vi "Test RPI Lib_SenseHat Display Register.vi"() -> ()   [LabVIEW 2020]
uses:
  <vilib>/MakerHub/LINX/Public/Utilities/Open Local.vi
  <vilib>/MakerHub/LINX/LMH-LINX.lvlib
  src/RPI/Classes/mainI2CDevice/mainI2CDevice.lvclass
panel:
  out "Data":u8[](array[numeric])
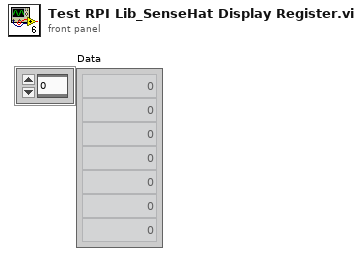
[diagram p1: front panel]
types:
  T1 = typedef "LMH-LINX.lvlib/LINX Ref.ctl" = cluster{"IO":T2, "Interface":T3, "LINX Device Config":T4}
  T2 = typedef "LMH-LINX.lvlib/Platform.ctl" = enum16{"Remote", "Local"}
  T3 = typedef "LMH-LINX.lvlib/Interface.ctl" = enum16{"Serial", "TCP"}
  T4 = typedef "LMH-LINX.lvlib/Device.lvlib/LINX Device Config.ctl" = cluster{"Interface":T3, "COM Port":refnum<visa-resource-name>, "TCP Configuration":T5, "Device Family":u8, "Device ID":u8, "Device Name":string, "TCP Ref":refnum<k5>, "Channels":T6}
  T5 = typedef "LMH-LINX.lvlib/Device.lvlib/TCP Config.ctl" = cluster{"IP Address":string, "Port":u16}
  T6 = typedef "LMH-LINX.lvlib/Channels.ctl" = cluster{"DI":u8[], "DO":u8[], "AI":u8[], "AO":u8[], "PWM":u8[], "QE":u8[], "UART":u8[], "I2C 2":u8[], "SPI":u8[], "CAN":u8[], "Servo":u8[], "AI Ref (V)":dbl, "AI Resolution (Bits)":u8, "AO Ref (V)":dbl, "AO Resolution (Bits)":u8}
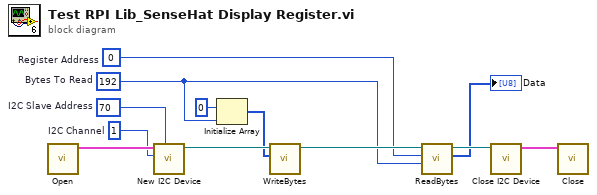
[diagram p0: block diagram]
diagram:
  w1 = u8 0  # Register Address
  w2 = u8 192  # Bytes To Read
  w9 = u8 70  # I2C Slave Address
  w10 = u8 1  # I2C Channel
  n1 = call-poly <vilib>:"Open.vi"() -> ("LINX Resource"=w12:T1)  [unwired: 9 in, 2 out]
  n2 = call "New I2C Device.vi"("I2C Slave Address"=w9, "I2C Channel"=w10, "object in"=w12) -> ("mainI2CDevice out"=w6:refnum<class "mainI2CDevice.lvclass">)  [unwired: 7 in, 1 out]
  n3 = Initialize Array(u8 0 ("element"), w2) -> (w4:u8[])
  n4 = call "WriteBytes.vi"("Data"=w4, "mainI2CDevice in"=w6) -> ("mainI2CDevice out"=w5:refnum<class "mainI2CDevice.lvclass">)  [unwired: 8 in, 1 out]
  n5 = call "ReadBytes.vi"("Bytes To Read"=w2, "Register Address"=w1, "mainI2CDevice in"=w5) -> ("Data"=→"Data":u8[], "mainI2CDevice out"=w8:refnum<class "mainI2CDevice.lvclass">)  [unwired: 6 in, 1 out]
  n6 = call "Close I2C Device.vi"("mainI2CDevice in"=w8) -> ("LINX Resource"=w11:T1)  [unwired: 9 in, 1 out]
  n7 = call <vilib>:"Close.vi"("LINX Resource"=w11) -> ()  [unwired: 10 in, 1 out]
